vi "InvokeMatlabMethod.vi"(7 "Invoke (t)?":bool=TRUE, 8 "error in (no error)":errorcluster, 9 "Arguments":variant, 10 "Method Name":string, 11 "ExpID":string) -> (0 "error out":errorcluster)   [LabVIEW 2017]
uses:
  Types/MethodInvokeInfo.ctl
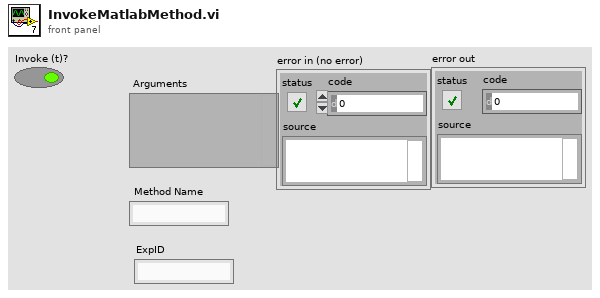
[diagram p1: front panel]
types:
  T1 = typedef "MethodInvokeInfo.ctl" = cluster{"Method Name":string, "Arguments":variant}
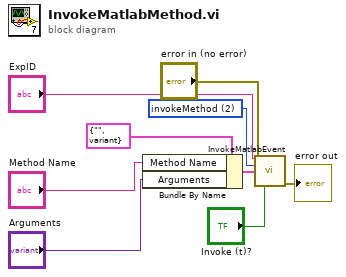
[diagram p0: block diagram]
diagram:
  w5 = u16 2 items=["[FromStringName]", "updateExpParameter", "invokeMethod"] ("Event")
  n1 = Bundle By Name(cluster=T1 {"Method Name"="", "Arguments"=variant}, "Method Name"="Method Name", "Arguments"="Arguments") -> (w7:T1)
  n2 = call "InvokeMatlabEvent.vi"("ExpID"="ExpID", "Event"=w5, "Data"=w7, "error in (no error)"="error in (no error)", "Invoke?"="Invoke (t)?") -> ("error out"=→"error out":errorcluster)  [unwired: 10 in]
